vi "Telnet_RW_wResp.vi"(5 "report_path":path, 6 "bytes to read (1024)":i32=1024, 7 "Delay Time (s)":dbl=0.3, 8 "error in (no error)":errorcluster, 9 "expected string":string, 10 "Write Telnet Command":string, 11 "connection ID":refnum<k5>) -> (0 "error out":errorcluster, 1 "String found?":bool, 2 "string out":string, 3 "connection ID out":refnum<k5>)   [LabVIEW 2018]
doc: "This VI sends a command using telnet and verifies the response is the expected one."
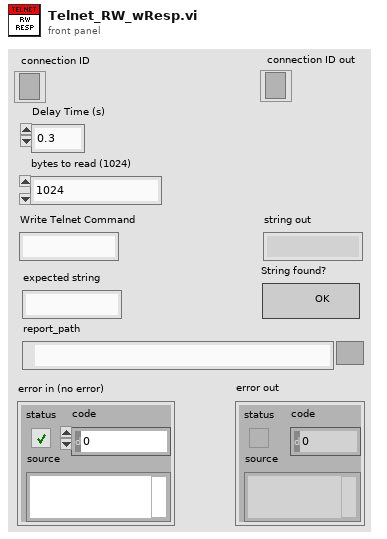
[diagram p1: front panel]
types:
  T1 = enum16{"Standard", "Buffered", "CRLF", "Immediate"}
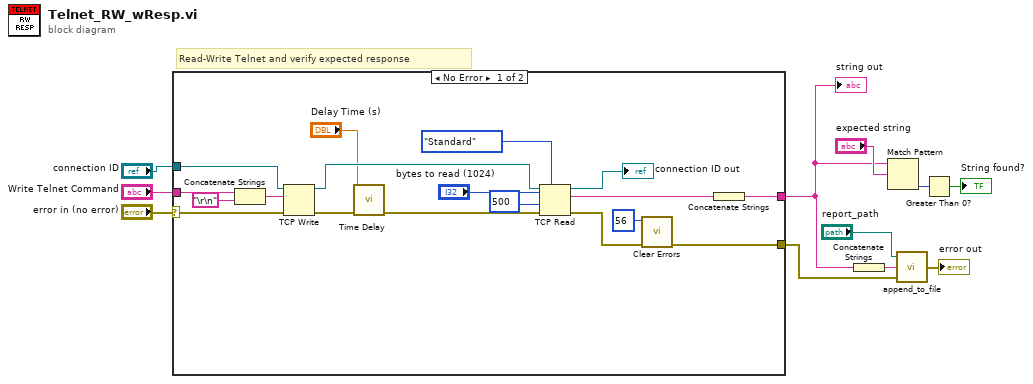
[diagram p0: block diagram]
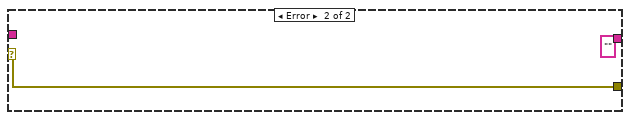
[diagram p2: hidden frame]
diagram:
  # "Read-Write Telnet and verify expected response"
  n1 = case shown="No Error" "error in (no error)" {
    selector: "error in (no error)" -> [w13 w30]
    tunnel: [w21 ""] -> w2
    tunnel: [w20 w30] -> w1
    tunnel: "Write Telnet Command" -> [w17 _]
    tunnel: "connection ID" -> [w14 _]
    frame No Error {
      n2 = Concatenate Strings(w17, "\r\n") -> (w19:string)
      n3 = TCP Write(connection ID=w14, data in=w19, error in (no error)=w13) -> (connection ID out=w16:refnum<k5>, error out=w15:errorcluster)  [unwired: 1 in, 1 out]
      n4 = call "Time Delay"("error in (no error)"=w15, "Delay Time (s)"="Delay Time (s)") -> ("error out"=w23:errorcluster)  [unwired: 9 in]
      n5 = TCP Read(connection ID=w16, bytes to read="bytes to read (1024)", error in (no error)=w23, 7:T1."Standard" ("mode (standard)"), 9:500 ("timeout ms (25000)")) -> (connection ID out=→"connection ID out":refnum<k5>, data out=w22:string, error out=w26:errorcluster)
      n6 = call "Clear Errors.vi"("error in (no error)"=w26, "specific error code to clear (0: all)"=56) -> ("error out"=w20:errorcluster)  [unwired: 4 in, 1 out]
      n7 = Concatenate Strings(w22) -> (w21:string)
    }
    frame Error {
    }
  }
  "string out" <- w2
  n8 = Concatenate Strings(w2) -> (w6:string)
  n9 = Match Pattern(string=w2, regular expression="expected string") -> (offset past match=w5:i32)  [unwired: 1 in, 3 out]
  n10 = call "append_to_file.vi"("error in (no error)"=w1, "text"=w6, "file_path"="report_path") -> ("error out"=→"error out":errorcluster)
  n11 = Greater Than 0?(x=w5) -> (x > 0?=→"String found?":bool)
